vi "CDS Placement Cleanup.vi"(8 "error in (no error)":errorcluster, 10 "Assert VI Ref":refnum<vi>, 11 "Assert VI Path":path) -> (0 "error out":errorcluster)   [LabVIEW 2018]
uses:
  207e34dd-bcd4-41c7-be6e-a9ed088be903.vi
  <vilib>/JDP Science/JSONtext/Find Item.vi
  207e34dd-bcd4-41c7-be6e-a9ed088be903.vi/db7a6e3f-78ed-4839-8f75-342cd1167dce.vi
  <vilib>/JDP Science/JSONtext/String Subset.vi
  Wizard Config/Wizard Strings.vi
  Wizard Config/Create Default Wizard Configuration.vi
  <vilib>/JDP Science/JSONtext/Parsing/Parse Full Path or Item Name.vi
  <vilib>/JDP Science/JSONtext/Offset/Find Item Locations by Path.vi
  <vilib>/JDP Science/JSONtext/JSON text to Variant.vi
  <vilib>/Utility/error.llb/Error Cluster From Error Code.vi
  <vilib>/ErrorRing/Error Ring.xnode
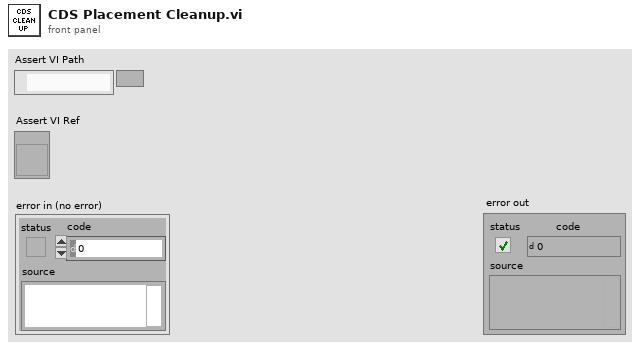
[diagram p1: front panel]
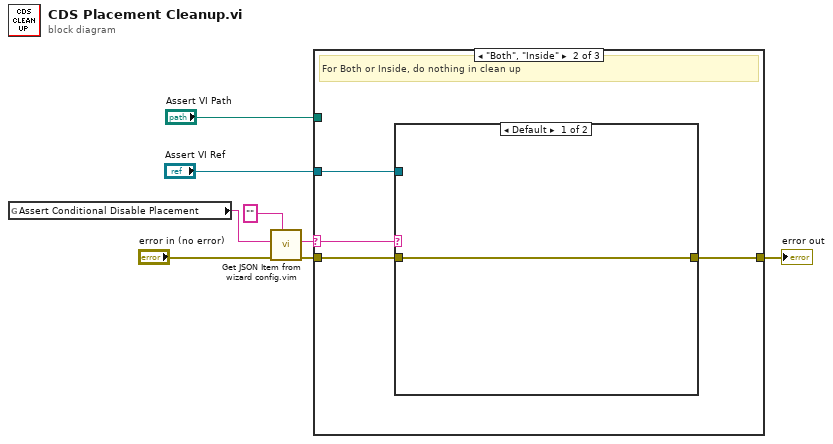
[diagram p0: block diagram]
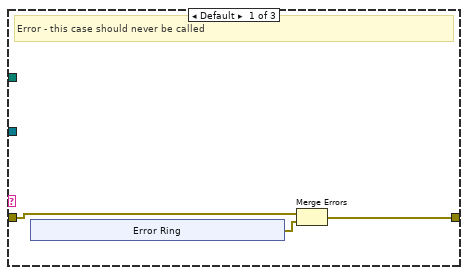
[diagram p2: hidden frame]
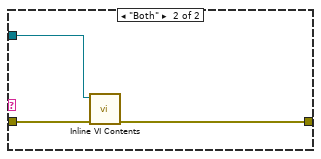
[diagram p3: hidden frame]
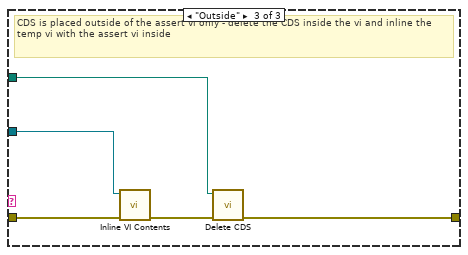
[diagram p4: hidden frame]
diagram:
  n1 = global read "Wizard Strings.vi" "Assert Conditional Disable Placement"() -> (w8:string)
  n2 = call "Get JSON Item from wizard config.vim"("Data Type"="" ("$Path or Item Name"), "error in (no error)"="error in (no error)", "$Path or Item Name"=w8) -> ("error out"=w4:errorcluster, "<JSON>"=w5:string)  [unwired: 6 in, 1 out]
  n3 = case shown="\"Both\", \"Inside\"" w5 {
    selector: w5 -> [_ w20 _]
    tunnel: w4 -> [w9 w19 w28]
    tunnel: [w10 w18 w27] -> w3
    tunnel: "Assert VI Path" -> [_ _ w29]
    tunnel: "Assert VI Ref" -> [_ w17 w25]
    frame Default {
      # "Error - this case should never be called"
      n4 = xnode "Error Ring"() -> ("error out"=w11:errorcluster)
      n5 = Merge Errors(w9, w11) -> (w10:errorcluster)
    }
    frame "Both", "Inside" {
      # "For Both or Inside, do nothing in clean up"
      n6 = case shown="Default" w20 {
        tunnel: w19 -> [w21 w24]
        tunnel: [w21 w23] -> w18
        tunnel: w17 -> [_ w22]
        frame Default {
        }
        frame "Both" {
          n7 = call "Inline VI Contents.vi"("error in (no error)"=w24, "SubVI in"=w22) -> ("error out"=w23:errorcluster)  [unwired: 9 in]
        }
      }
    }
    frame "Outside" {
      # "CDS is placed outside of the assert vi only - delete the CDS inside the vi and inline the temp vi with the assert vi inside"
      n8 = call "Inline VI Contents.vi"("error in (no error)"=w28, "SubVI in"=w25) -> ("error out"=w26:errorcluster)  [unwired: 9 in]
      n9 = call "Delete CDS.vi"("error in (no error)"=w26, "Assert VI Path"=w29) -> ("error out"=w27:errorcluster)  [unwired: 8 in, 1 out]
    }
  }
  "error out" <- w3
